vi "PSK调制与解调.vi"() -> ()   [LabVIEW 2013]
uses:
  <vilib>/measure/maspectr.llb/FFT Spectrum (Mag-Phase) for 1 Chan.vi
  <vilib>/Analysis/3filter.llb/Butterworth Filter (DBL).vi
  <vilib>/measure/NI_MAPro.lvlib
  <vilib>/Analysis/NI_AALBase.lvlib
panel:
  out "滤波后波形":dbl[](graph)
  out "2PSK频谱图":cluster{"f0":dbl, "df":dbl, "magnitude":dbl[]}(graph)
  out "2PSK信号波形":dbl[](graph)
  out "载波波形2":dbl[](graph)
  out "载波波形1":dbl[](graph)
  out "输入序列波形":dbl[](graph)
  out "一个码周期内的点数":dbl
  in  "码速率":dbl
  in  "载频":dbl
  in  "载波相位":dbl
  in  "采样率":dbl
  in  "采样点数":i32
  out "输出序列":u32[](array[numeric])
  in  "输入序列":u32[](array[numeric]) format="%b"
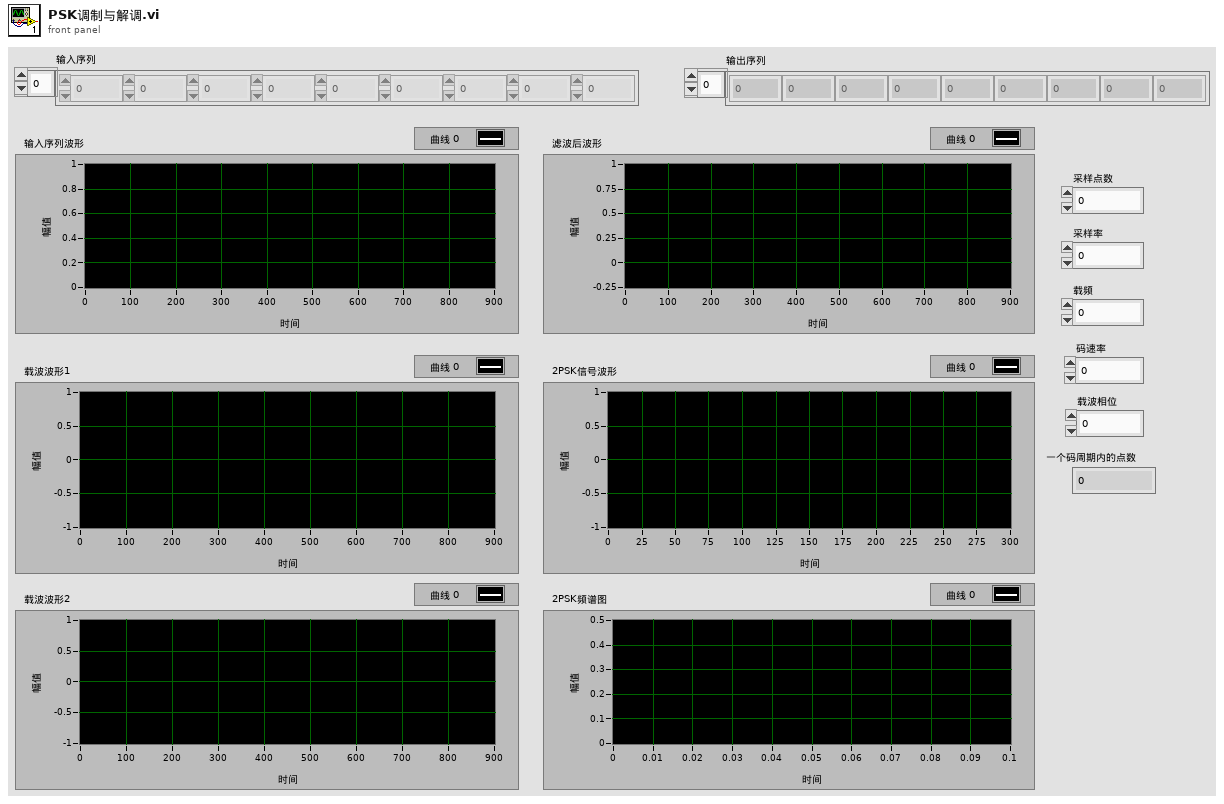
[diagram p1: front panel]
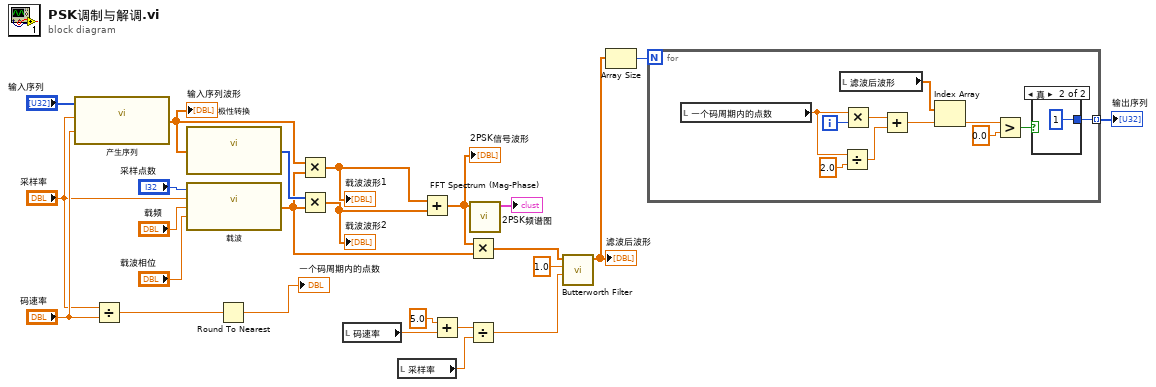
[diagram p0: block diagram]
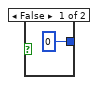
[diagram p2: hidden frame]
diagram:
  n1 = call "产生序列.vi"("码速率RB"="码速率", "采样率"="采样率", "输入序列"="输入序列") -> ("输入序列波形"=w13:dbl[])
  "输入序列波形" <- w13
  n2 = Divide(x="采样率", y="码速率") -> (x/y=w19:dbl)
  n3 = call "极性转换.vi"("1、0码"=w13) -> ("0、-1码"=w14:i32[])
  n4 = call "载波.vi"("相位输入"="载波相位", "载频"="载频", "采样率"="采样率", "采样点数"="采样点数") -> ("载波信号波形"=w9:dbl[])
  n5 = Round To Nearest(number=w19) -> (nearest integer value=→"一个码周期内的点数":dbl)
  n6 = Multiply(x=w13, y=w9) -> (x*y=w12:dbl[])
  "载波波形1" <- w12
  n7 = Multiply(x=w14, y=w9) -> (x*y=w11:dbl[])
  "载波波形2" <- w11
  n8 = local read "码速率"() -> (w7:dbl)
  n9 = local read "采样率"() -> (w5:dbl)
  n10 = Add(x=w12, y=w11) -> (x+y=w10:dbl[])
  "2PSK信号波形" <- w10
  n11 = Add(x=5.0, y=w7) -> (x+y=w6:dbl)
  n12 = Multiply(x=w10, y=w9) -> (x*y=w2:dbl[])
  n13 = Divide(x=w6, y=w5) -> (x/y=w4:dbl)
  n14 = call-poly <vilib>:"FFT Spectrum (Mag-Phase).vi"("time signal"=w10) -> ("magnitude"=→"2PSK频谱图":cluster{"f0":dbl, "df":dbl, "magnitude":dbl[]})  [unwired: 6 in, 4 out]
  n15 = call-poly <vilib>:"Butterworth Filter.vi"("high cutoff freq: fh"=w4, "sampling freq: fs"=1.0, "X"=w2) -> ("Filtered X"=w1:dbl[])  [unwired: 5 in, 1 out]
  "滤波后波形" <- w1
  n16 = Array Size(array=w1) -> (size(s)=w16:i32)
  n17 = for {
    N: w16 -> [_]
    tunnel: [w31] -> w15 mode=indexing
    i -> [w36]
    n18 = local read "一个码周期内的点数"() -> (w33:dbl)
    n19 = local read "滤波后波形"() -> (w28:dbl[])
    n20 = Divide(x=w33, y=2.0) -> (x/y=w34:dbl)
    n21 = Multiply(x=w33, y=w36) -> (x*y=w30:dbl)
    n22 = Add(x=w30, y=w34) -> (x+y=w29:dbl)
    n23 = Index Array(array=w28, index=w29) -> (element=w26:dbl)
    n24 = Greater?(x=w26, y=0.0) -> (0:w32:bool)
    n25 = case shown="真" w32 {
      tunnel: [0 1] -> w31
      frame False {
      }
      frame True {
      }
    }
  }
  "输出序列" <- w15
